vi "Cross-Talk, Determine Off Channel.vi"(8 "error in":errorcluster, 9 "Resistance (ohms)":dbl, 10 "Target Amplitude (mA)":dbl, 11 "Waveform":waveform(dbl)) -> (0 "error out":errorcluster, 3 "Off Channel?":bool)   [LabVIEW 2010]
uses:
  <vilib>/measure/mamon.llb/Trigger Detection for 1 Channel.vi
  <vilib>/measure/NI_MAPro.lvlib
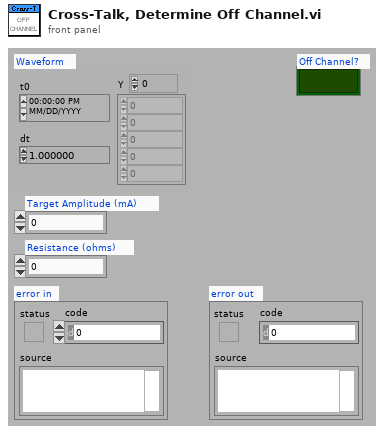
[diagram p1: front panel]
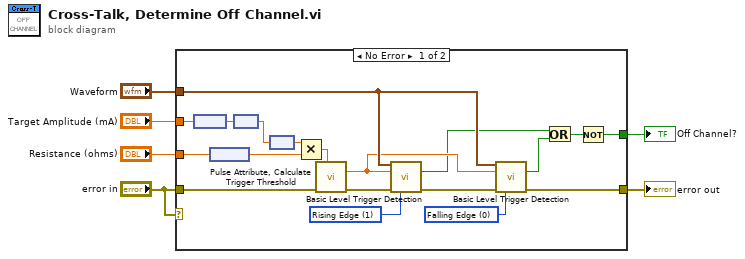
[diagram p0: block diagram]
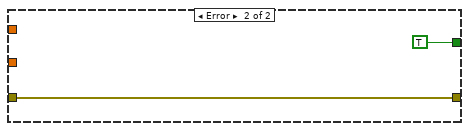
[diagram p2: hidden frame]
diagram:
  n1 = case shown="No Error" "error in" {
    tunnel: "Waveform" -> [w25 _]
    tunnel: [w24 w27] -> w5
    tunnel: "Target Amplitude (mA)" -> [w9 _]
    tunnel: "Resistance (ohms)" -> [w12 _]
    tunnel: "error in" -> [w20 w27]
    tunnel: [w14 TRUE] -> w2
    frame No Error {
      w21 = u16 0 items=["Falling Edge", "Rising Edge"] ("trigger slope")
      w22 = u16 1 items=["Falling Edge", "Rising Edge"] ("trigger slope")
      n2 = node(w9) -> (w10:dbl[unit])
      n3 = node(w12) -> (w13:dbl[unit])
      n4 = node(w10) -> (w8:dbl)
      n5 = node(w8) -> (w7:dbl[unit])
      n6 = Multiply(x=w7, y=w13) -> (x*y=w11:dbl[unit])
      n7 = call "Pulse Attribute, Calculate Trigger Threshold.vi"("pulse amp"=w11, "error in"=w20) -> ("error out"=w19:errorcluster, "trigger level (V)"=w18:dbl)  [unwired: 5 in]
      n8 = call-poly <vilib>:"Basic Level Trigger Detection.vi"("signal in"=w25, "level"=w18, "error in (no error)"=w19, "trigger slope"=w22) -> ("trigger detected?"=w17:bool, "error out"=w23:errorcluster)  [unwired: 9 in, 1 out]
      n9 = call-poly <vilib>:"Basic Level Trigger Detection.vi"("signal in"=w25, "level"=w18, "error in (no error)"=w23, "trigger slope"=w21) -> ("trigger detected?"=w16:bool, "error out"=w24:errorcluster)  [unwired: 9 in, 1 out]
      n10 = Or(x=w17, y=w16) -> (x .or. y?=w15:bool)
      n11 = Not(x=w15) -> (.not. x?=w14:bool)
    }
    frame Error {
    }
  }
  "error out" <- w5
  "Off Channel?" <- w2
